vi "Keithley 2400 - Read.vi"(11 "Porta:":refnum<visa-resource-name>="COM5") -> (0 "Corrente:":dbl, 3 "Tensão:":dbl)   [LabVIEW 2017]
uses:
  <vilib>/Instr/_visa.llb/VISA Configure Serial Port (Instr).vi
panel:
  out "error out":errorcluster
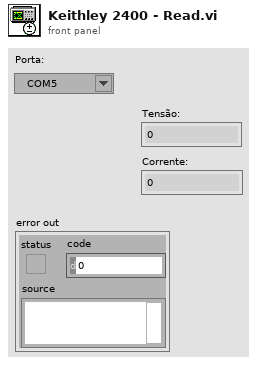
[diagram p1: front panel]
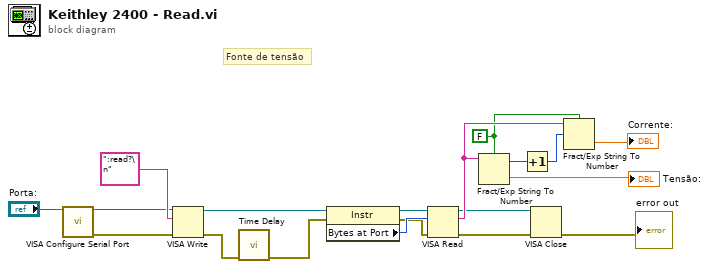
[diagram p0: block diagram]
diagram:
  w5 = FALSE ("use system decimal point (T)")
  # "Fonte de tensão"
  n1 = call-poly "VISA Configure Serial Port"("VISA resource name"="Porta:") -> ("VISA resource name out"=w2:refnum<visa-resource-name>, "error out"=w1:errorcluster)  [unwired: 13 in]
  n2 = VISA Write(VISA resource name=w2, write buffer=":read?\n", error in (no error)=w1) -> (VISA resource name out=w15:refnum<visa-resource-name>, error out=w17:errorcluster)  [unwired: 1 out]
  n3 = call "Time Delay"("error in (no error)"=w17) -> ("error out"=w16:errorcluster)  [unwired: 10 in]
  n4 = property class="Instr"(reference=w15, error in=w16) -> (reference out=w13:refnum<visa-resource-name>, error out=w12:errorcluster, "Bytes at Port"=w14:u32)
  n5 = VISA Read(VISA resource name=w13, byte count=w14, error in (no error)=w12) -> (VISA resource name out=w4:refnum<visa-resource-name>, read buffer=w10:string, error out=w3:errorcluster)  [unwired: 1 out]
  n6 = Fract/Exp String To Number(use system decimal point (T)=w5, string=w10) -> (offset past number=w9:i32, number=→"Tensão:":dbl)  [unwired: 2 in]
  n7 = Increment(x=w9) -> (x+1=w8:i32)
  n8 = VISA Close(VISA resource name=w4, error in (no error)=w3) -> (error out=→"error out":errorcluster)
  n9 = Fract/Exp String To Number(use system decimal point (T)=w5, string=w10, offset=w8) -> (number=→"Corrente:":dbl)  [unwired: 1 in, 1 out]
